vi "MeasureInstr.vi"(1 "Measure Current?":bool, 8 "error in (no error)":errorcluster, 11 "Device reference":refnum<class "Device.lvclass">) -> (0 "error out":errorcluster, 2 "Data":waveform(dbl)[](array[waveform]), 3 "Device reference out":refnum<class "Device.lvclass">)   [LabVIEW 2015]
uses:
  OO Devices/Device/Device.lvclass
panel:
  out "Actual Current":dbl format="%.3e"
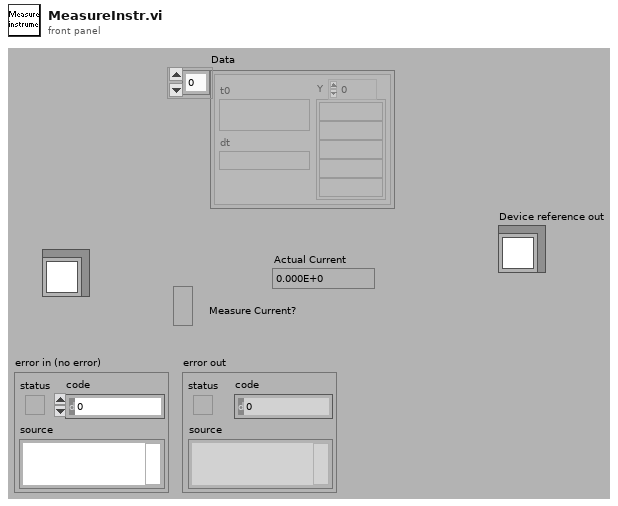
[diagram p1: front panel]
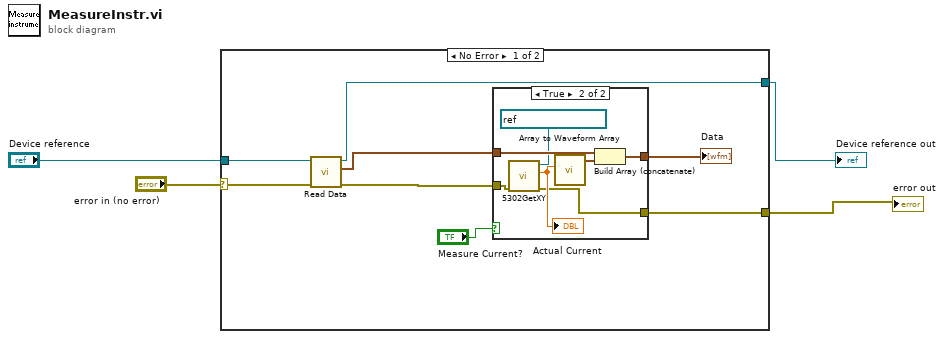
[diagram p0: block diagram]
diagram:
  n1 = case shown="No Error" "error in (no error)" {
    selector: "error in (no error)" -> [w6 w22]
    tunnel: [w11 w22] -> w2
    tunnel: "Device reference" -> [w8 w23]
    tunnel: [w5 w23] -> w3
    frame No Error {
      n2 = call-dynamic "Read Data.vi"("error in (no error)"=w6, "Device in"=w8) -> ("error out"=w10:errorcluster, "Data"=w9:waveform(dbl)[], "Device out"=w5:refnum<class "Device.lvclass">)  [unwired: 7 out]
      n3 = case shown="True" "Measure Current?" {
        tunnel: w9 -> [w14 w21]
        tunnel: [w14 w20] -> w7
        tunnel: w10 -> [w13 w18]
        tunnel: [w13 w17] -> w11
        frame False {
        }
        frame True {
          n4 = call "5302GetXY.vi"("error in (no error)"=w18, "VISA Resource Name"=refnum<visa-resource-name> "GPIB0:6::INSTR") -> ("error out"=w17:errorcluster, "X"=w19:dbl)  [unwired: 1 in, 7 out]
          "Actual Current" <- w19
          n5 = call "Array to Waveform Array.vi"("dt"=w19) -> ("Waveform"=w15:waveform(dbl)[])  [unwired: 10 in]
          n6 = Build Array (concatenate)(w21, w15) -> (w20:waveform(dbl)[])
        }
      }
      "Data" <- w7
    }
    frame Error {
    }
  }
  "error out" <- w2
  "Device reference out" <- w3
